vi "remove-dev-pointsSD.vi"(1 "IN data lamda at ceratin time":dbl[](array[numeric])) -> (0 "Average without bad points":dbl)   [LabVIEW 2015]
uses:
  <vilib>/Analysis/6fits.llb/Remove Outliers (Range).vi
  <vilib>/Analysis/baseanly.llb/Mean (DBL).vi
  globalVarSD.vi
  <vilib>/Analysis/NI_AALBase.lvlib
  <vilib>/Analysis/NI_AALPro.lvlib
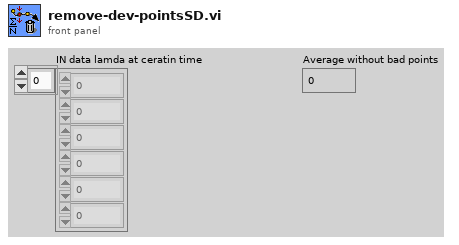
[diagram p1: front panel]
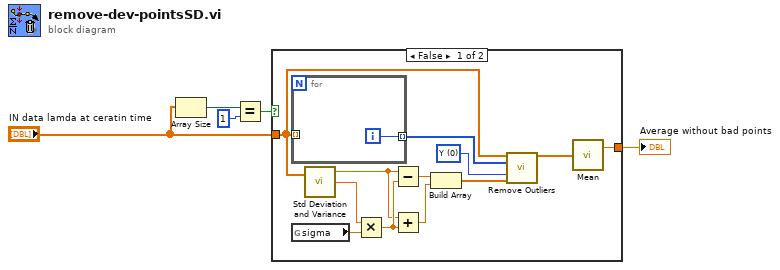
[diagram p0: block diagram]
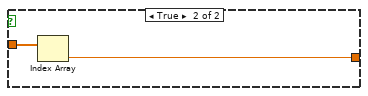
[diagram p2: hidden frame]
diagram:
  n1 = Array Size(array="IN data lamda at ceratin time") -> (size(s)=w3:i32)
  n2 = Equal?(x=w3, y=1) -> (x = y?=w1:bool)
  n3 = case shown="False" w1 {
    tunnel: "IN data lamda at ceratin time" -> [w13 w20]
    tunnel: [w8 w19] -> w5
    frame False {
      w12 = u16 0 items=["Y", "X", "X et Y"] ("range type")
      n4 = for {
        tunnel: [w18] -> w14 mode=indexing
        tunnel: w13 -> [_] mode=indexing
        i -> [w18]
      }
      n5 = global read "globalVarSD.vi" "sigma"() -> (w6:dbl)
      n6 = call <vilib>:"Std Deviation and Variance.vi"("X"=w13) -> ("mean"=w15:dbl, "standard deviation"=w16:dbl)  [unwired: 1 in, 1 out]
      n7 = Multiply(x=w16, y=w6) -> (x*y=w17:dbl)
      n8 = Subtract(x=w15, y=w17) -> (x-y=w10:dbl)
      n9 = Add(x=w15, y=w17) -> (x+y=w11:dbl)
      n10 = Build Array(w10, w11) -> (w9:dbl[])
      n11 = call-poly <vilib>:"Remove Outliers.vi"("Y"=w13, "X"=w14, "range type"=w12, "Range"=w9) -> ("Y Out"=w7:dbl[])  [unwired: 7 in, 4 out]
      n12 = call-poly <vilib>:"Mean.vi"("X"=w7) -> ("mean"=w8:dbl)  [unwired: 1 out]
    }
    frame True {
      n13 = Index Array(array=w20) -> (element=w19:dbl)  [unwired: 1 in]
    }
  }
  "Average without bad points" <- w5
